vi "Write.vi"(8 "error in (no error)":errorcluster, 11 "navX - Base in":refnum<class "navX - Base.lvclass">) -> (0 "error out":errorcluster, 3 "navX - Base out":refnum<class "navX - Base.lvclass">)   [LabVIEW 2015, in "navX Library v3.lvlib" / "navX - Base.lvclass"]
uses:
  navX - Base.lvclass
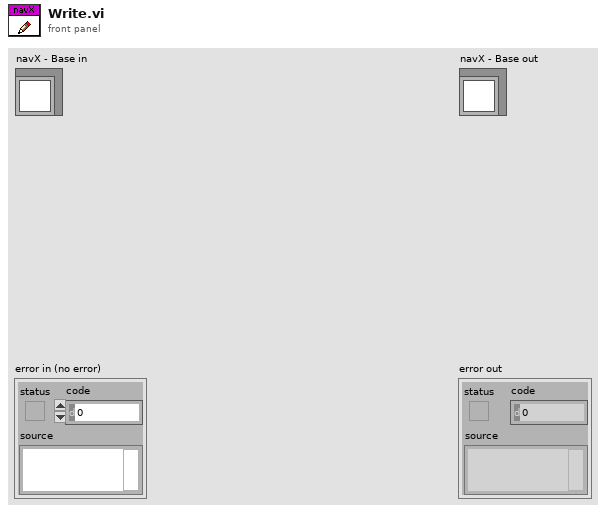
[diagram p1: front panel]
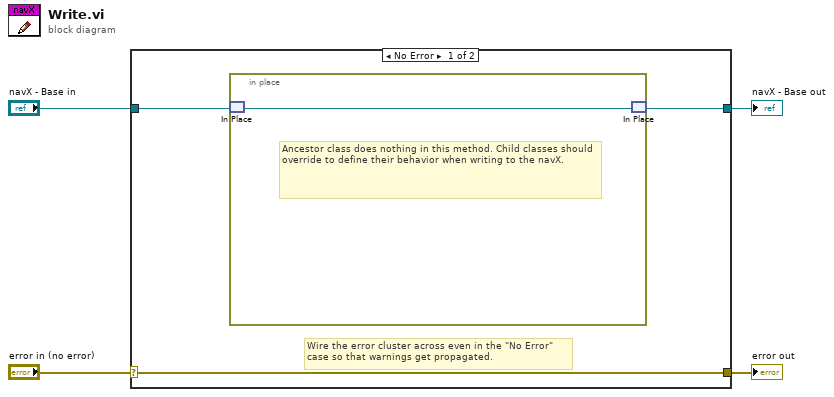
[diagram p0: block diagram]
diagram:
  n1 = case shown="No Error" "error in (no error)" {
    selector: "error in (no error)" -> [w7 w10]
    tunnel: [w7 w10] -> w3
    tunnel: [w5 w9] -> w1
    tunnel: "navX - Base in" -> [w6 w9]
    frame No Error {
      # "Wire the error cluster across even in the \"No Error\"\ncase so that warnings get propagated."
      n2 = in-place {
        # "Ancestor class does nothing in this method. Child classes should override to define their behavior when writing to the navX."
        n3 = in-place-match #1(w6) -> (w8:refnum<class "navX - Base.lvclass">)
        n4 = in-place-match #1(w8) -> (w5:refnum<class "navX - Base.lvclass">)
      }
    }
    frame Error {
    }
  }
  "error out" <- w3
  "navX - Base out" <- w1
